vi "StdDev vs ApertureTime.vi"(4 "Source:Advanced:Source Delay":dbl=4e-05 format="%#_6p", 5 "Source:Transient Response":i32(ring)=1039 items=["Slow"=1041, "Normal"=1038, "Fast"=1039, "Custom"=1042], 7 "Measurement:Sense":i32(ring)=1009 items=["Local"=1008, "Remote"=1009], 8 "channels":string="0", 9 "Current":dbl=0.4 format="%#_6p", 10 "Voltage":dbl=0.6 format="%#_6p", 11 "resource name":refnum<k15>="SMU") -> (2 "R":dbl=3.092139974281396e-05 format="%#_8p")   [LabVIEW 2018]
uses:
  <instrlib>/niDCPower/nidcpower.llb/niDCPower Wait For Event - Event.ctl
  <vilib>/ptbypt/NI_PtbyPt.lvlib
panel:
  out "Standard Deviation (Ohm)":dbl[](array[numeric])=[2.747699345089886e-07, 1.2829614567464684e-07, 1.252678452782734e-07, 9.046214015260652e-08, 9.119373094920907e-08, 8.70740018095382e-08, 7.254873375422988e-08, 6.78166950902716e-08] format="%#_6p"
  out "Aperture Time (s)":dbl[](array[numeric])=[0.0166666666666667, 0.0333333333333333, 0.05, 0.0666666666666667, 0.0833333, 0.1, 0.166667, 0.333333] format="%#_6p"
  out "Standard Deviation (Ohm) vs Aperture Time (s)":cluster{"Y":dbl[], "Y":dbl[]}[](graph)=[{"Y"=[0.0166666666666667, 0.0333333333333333, 0.05, 0.0666666666666667, 0.0833333, 0.1, 0.166667, 0.333333], "Y"=[2.747699345089886e-07, 1.2829614567464684e-07, 1.252678452782734e-07, 9.046214015260652e-08, 9.119373094920907e-08, 8.70740018095382e-08, 7.254873375422988e-08, 6.78166950902716e-08]}]
  in  "Aperture Time":dbl[](array[numeric])=[0.0166666666666667, 0.0333333333333333, 0.05, 0.0666666666666667, 0.0833333, 0.1, 0.166667, 0.333333] format="%#_6p"
  out "error out":errorcluster
  out "current measurements":dbl[](array[numeric])=[0.4000000256132281, -0.399999965959666, -1.4913390512100166e-08]
  out "voltage measurements":dbl[](array[numeric])=[5.6648894241039145e-05, 3.1911774707365885e-05, 4.437444308112368e-05]
  in  "Measurement:Advanced:DC Noise Rejection":i32(ring)=1044 items=["Normal"=1044, "Second-Order"=1043]
  in  "Source:Advanced:Sequence Loop Count":i32=100
  out "standard deviation":dbl=6.78166950902716e-08 format="%.6p"
  out "Waveform Chart":dbl(graph)=3.092139974281396e-05
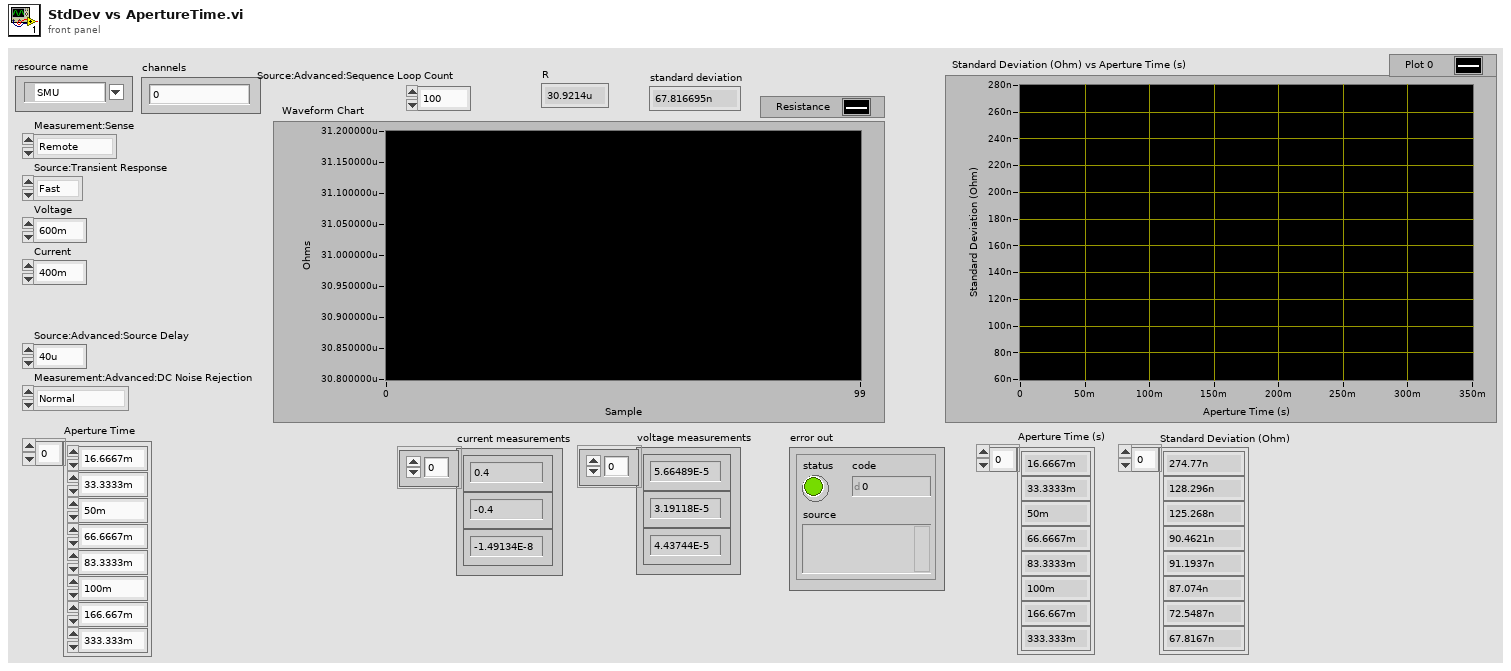
[diagram p1: front panel]
types:
  T1 = typedef "niDCPower Wait For Event - Event.ctl" = i32
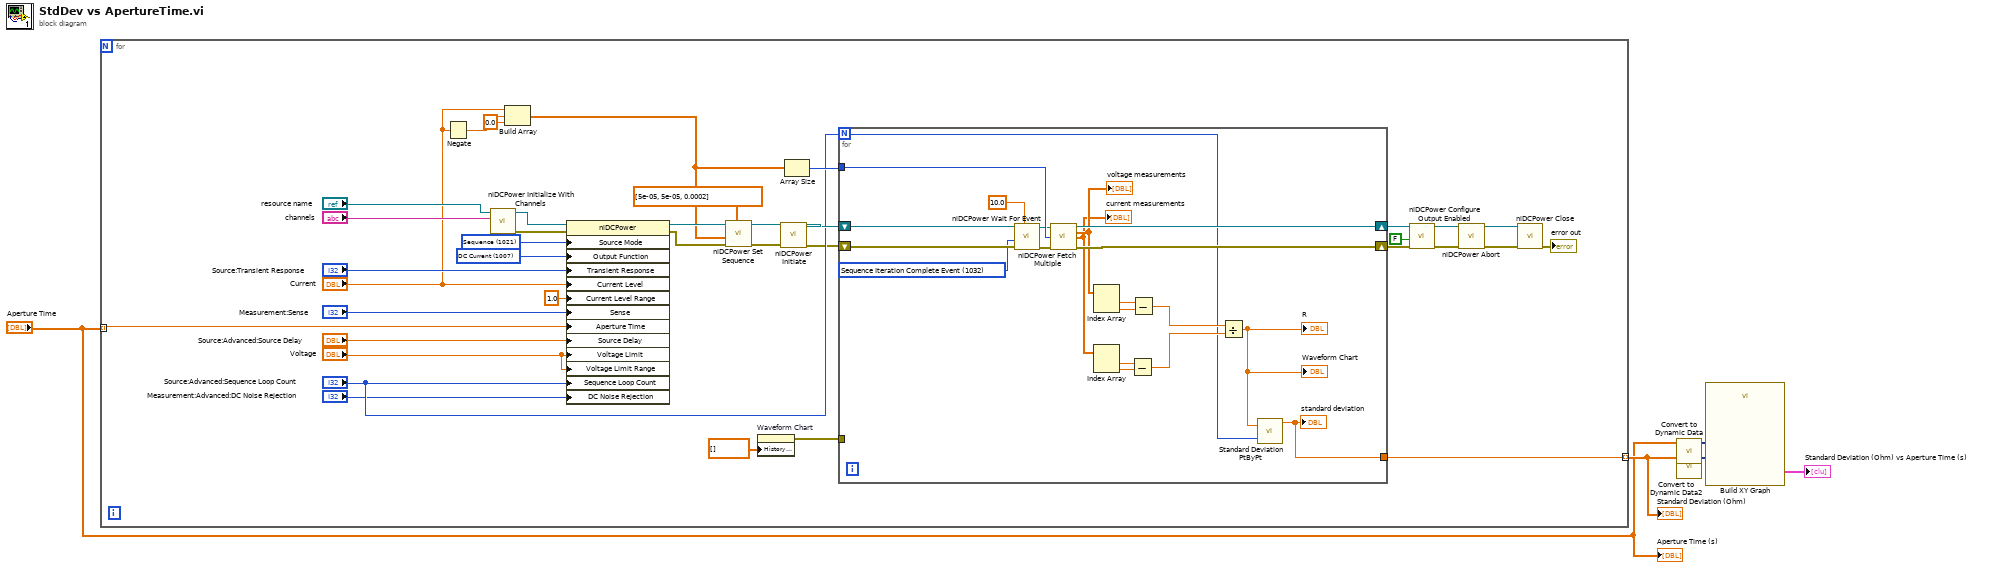
[diagram p0: block diagram]
diagram:
  n1 = for {
    tunnel: "Aperture Time" -> [w7] mode=indexing
    tunnel: [w6] -> w2 mode=indexing
    w41 = 1007 items=["DC Voltage"=1006, "DC Current"=1007, "Pulse Voltage"=1049, "Pulse Current"=1050] ("Source:Output Function")
    w42 = 1021 items=["Single Point"=1020, "Sequence"=1021] ("Source:Source Mode")
    n2 = Negate(x="Current") -> (-x=w33:dbl)
    n3 = call <instrlib>:"niDCPower Initialize With Channels.vi"("channels"="channels", "resource name"="resource name") -> ("error out"=w28:errorcluster, "instrument handle out"=w29:refnum<k15>)  [unwired: 8 in]
    n4 = Build Array("Current", w33, 0.0 ("element")) -> (w32:dbl[])
    n5 = property class="niDCPower"(reference=w29, error in=w28, "Source Mode"=w42, "Output Function"=w41, "Transient Response"="Source:Transient Response", "Current Level"="Current", "Current Level Range"=1.0 ("Source:DC Current:Current Level Range"), "Sense"="Measurement:Sense", "Aperture Time"=w7, "Source Delay"="Source:Advanced:Source Delay", "Voltage Limit"="Voltage", "Voltage Limit Range"="Voltage", "Sequence Loop Count"="Source:Advanced:Sequence Loop Count", "DC Noise Rejection"="Measurement:Advanced:DC Noise Rejection") -> (reference out=w37:refnum<k15>, error out=w38:errorcluster)
    n6 = call <instrlib>:"niDCPower Set Sequence.vi"("source delays"=dbl[] [5e-05, 5e-05, 0.0002], "error in (no error)"=w38, "values"=w32, "instrument handle"=w37) -> ("error out"=w10:errorcluster, "instrument handle out"=w35:refnum<k15>)  [unwired: 6 in]
    n7 = property on="Waveform Chart" class="WFChart (strict)"("History Data"=dbl[] []) -> (error out=w21:errorcluster)  [unwired: 2 in, 1 out]
    n8 = call <instrlib>:"niDCPower Initiate.vi"("error in (no error)"=w10, "instrument handle"=w35) -> ("error out"=w9:errorcluster, "instrument handle out"=w25:refnum<k15>)  [unwired: 8 in]
    n9 = Array Size(array=w32) -> (size(s)=w34:i32)
    n10 = for {
      N: "Source:Advanced:Sequence Loop Count" -> [w44]
      tunnel: w34 -> [w62]
      shift-right: [w54] -> w17
      shift-left: w9 -> [w61]
      shift-right: [w55] -> w18
      shift-left: w25 -> [w60]
      tunnel: w21 -> [_]
      tunnel: [w43] -> w6
      w59 = T1 1032 items=["Source Complete Event"=1030, "Measure Complete Event"=1031, "Sequence Iteration Complete Event"=1032, "Sequence Engine Done Event"=1033, "Pulse Complete Event"=1051, "Ready For Pulse Trigger Event"=1052] ("event")
      n11 = call <instrlib>:"niDCPower Wait For Event.vi"("timeout (sec)"=10.0, "error in (no error)"=w61, "event"=w59, "instrument handle"=w60) -> ("error out"=w56:errorcluster, "instrument handle out"=w57:refnum<k15>)  [unwired: 6 in]
      n12 = call <instrlib>:"niDCPower Fetch Multiple.vi"("instrument handle"=w57, "count (1)"=w62, "error in (no error)"=w56) -> ("instrument handle out"=w55:refnum<k15>, "voltage measurements"=w53:dbl[], "current measurements"=w52:dbl[], "error out"=w54:errorcluster)  [unwired: 7 in, 2 out]
      "voltage measurements" <- w53
      "current measurements" <- w52
      n13 = Index Array(array=w53) -> (element #1=w51:dbl, element #2=w50:dbl)  [unwired: 2 in]
      n14 = Index Array(array=w52) -> (element #1=w48:dbl, element #2=w49:dbl)  [unwired: 2 in]
      n15 = Subtract(x=w48, y=w49) -> (x-y=w46:dbl)
      n16 = Subtract(x=w51, y=w50) -> (x-y=w47:dbl)
      n17 = Divide(x=w47, y=w46) -> (x/y=w45:dbl)
      "R" <- w45
      "Waveform Chart" <- w45
      n18 = call <vilib>:"Standard Deviation PtByPt.vi"("x"=w45, "sample length"=w44) -> ("standard deviation"=w43:dbl)  [unwired: 1 in, 2 out]
      "standard deviation" <- w43
    }
    n19 = call <instrlib>:"niDCPower Configure Output Enabled.vi"("error in (no error)"=w17, "output enabled"=FALSE, "instrument handle"=w18) -> ("error out"=w20:errorcluster, "instrument handle out"=w19:refnum<k15>)  [unwired: 7 in]
    n20 = call <instrlib>:"niDCPower Abort.vi"("error in (no error)"=w20, "instrument handle"=w19) -> ("error out"=w31:errorcluster, "instrument handle out"=w30:refnum<k15>)  [unwired: 8 in]
    n21 = call <instrlib>:"niDCPower Close.vi"("error in (no error)"=w31, "instrument handle"=w30) -> ("error out"=→"error out":errorcluster)  [unwired: 9 in]
  }
  "Standard Deviation (Ohm)" <- w2
  n22 = call "Convert to Dynamic Data"("Array"="Aperture Time") -> ("Dynamic Data Type"=w4:dynamicdata)  [unwired: 3 in]
  n23 = call "Convert to Dynamic Data2"("Array"=w2) -> ("Dynamic Data Type"=w3:dynamicdata)  [unwired: 3 in]
  n24 = call "Build XY Graph"("Y Input"=w3, "X Input"=w4) -> ("XY Graph"=→"Standard Deviation (Ohm) vs Aperture Time (s)":cluster{"X":dbl[], "Y":dbl[]}[])  [unwired: 8 in, 1 out]
  "Aperture Time (s)" <- "Aperture Time"
